vi "Run.vi"(8 "error in (no error)":errorcluster, 10 "TestResult":refnum<class "TestResult.lvclass">, 11 "TestCase in":refnum<class "TestCase.lvclass">) -> (0 "error out":errorcluster, 2 "TestResult out":refnum<class "TestResult.lvclass">, 3 "TestCase out":refnum<class "TestCase.lvclass">)   [LabVIEW 2019, in "TestCase.lvlib" / "TestCase.lvclass"]
doc: "Runs the test case and collects the results in a <B>TestResult</B> object."
uses:
  TestCase.lvclass
  TestResult/TestResult.lvclass
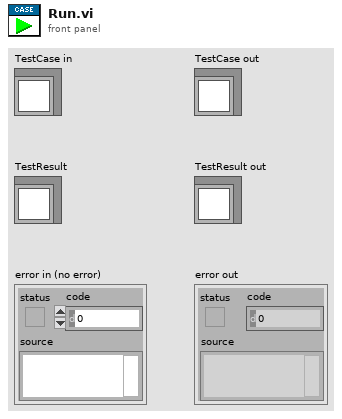
[diagram p1: front panel]
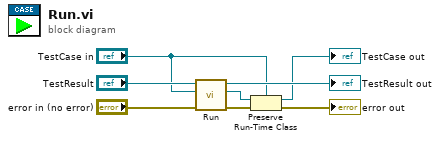
[diagram p0: block diagram]
diagram:
  n1 = call-dynamic "Run.vi"("error in (no error)"="error in (no error)", "TestCase"="TestCase in", "TestResult in"="TestResult") -> ("error out"=w5:errorcluster, "TestCase out"=w3:refnum<class "TestCase.lvclass">, "TestResult out"=→"TestResult out":refnum<class "TestResult.lvclass">)  [unwired: 6 in]
  n2 = Preserve Run-Time Class(object in=w3, error in=w5, 2:"TestCase in") -> (object out=→"TestCase out":refnum<class "TestCase.lvclass">, error out=→"error out":errorcluster)
